vi "Recipe.vi"() -> ()   [LabVIEW 2015]
panel:
  in  "Timer":bool
  in  "Offset":bool
  in  "Speed":bool
  in  "檔案":bool
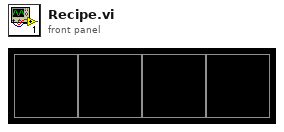
[diagram p1: front panel]
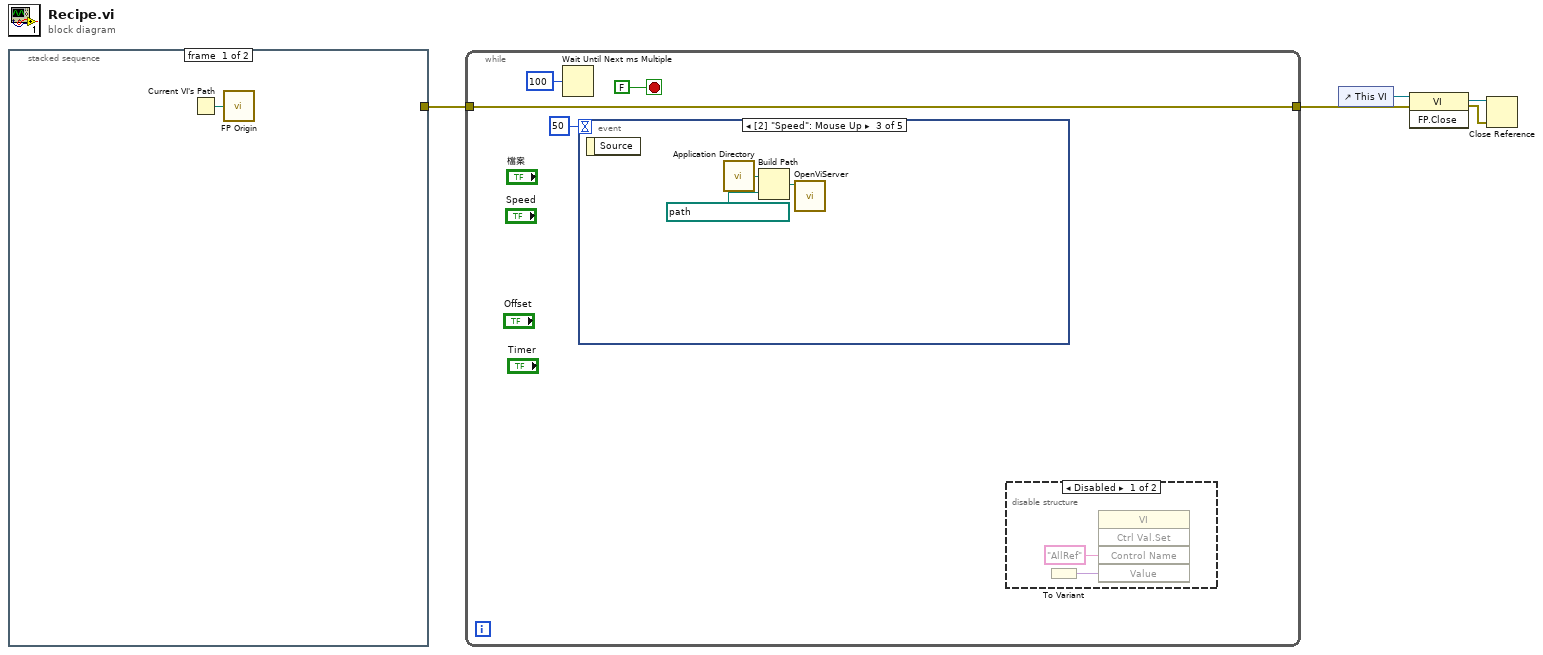
[diagram p0: block diagram]
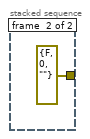
[diagram p2: hidden frame]
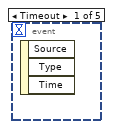
[diagram p4: hidden frame]
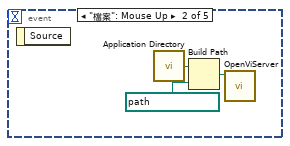
[diagram p5: hidden frame]
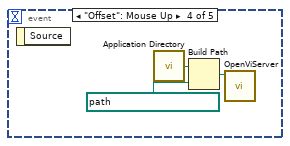
[diagram p6: hidden frame]
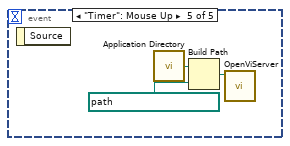
[diagram p7: hidden frame]
diagram:
  n1 = stacked-sequence {
    tunnel: [_ errorcluster {"status"=FALSE, "code"=0, "source"=""} ("error out")] -> w1
    frame #0 {
      n2 = Current VI's Path() -> (path=w6:path)
      n3 = call "FP Origin.vi"("vi path"=w6) -> ()  [unwired: 1 out]
    }
    frame #1 {
    }
  }
  n4 = while {
    tunnel: w1 -> [w9]
    tunnel: [w9] -> w5
    stop <- FALSE stop-if-true
    n5 = Wait Until Next ms Multiple(millisecond multiple=u32 100) -> ()  [unwired: 1 out]
    n6 = event shown="[2] \"Speed\": Mouse Up" {
      selector: _ -> [_ _ _ _ _]
      dyn-events: _ -> [_ _ _ _ _]
      timeout: 50 -> [_ _ _ _ _]
      event Timeout {
        n7 = event-data() -> ()  [unwired: 1 in, 3 out]
      }
      event "檔案": Mouse Up {
        n8 = event-data() -> ()  [unwired: 1 in, 1 out]
        n9 = call <vilib>:"Application Directory.vi"() -> ("Application Directory"=w15:path)
        n10 = Build Path(base path=w15, name or relative path=path "0.Main/檔案.vi" ("vi path")) -> (appended path=w17:path)
        n11 = call "OpenViServer.vi"("vi path"=w17) -> ()  [unwired: 9 in, 2 out]
      }
      event "Speed": Mouse Up {
        n12 = event-data() -> ()  [unwired: 1 in, 1 out]
        n13 = call <vilib>:"Application Directory.vi"() -> ("Application Directory"=w18:path)
        n14 = Build Path(base path=w18, name or relative path=path "0.Main/檔案_速度.vi" ("vi path")) -> (appended path=w20:path)
        n15 = call "OpenViServer.vi"("vi path"=w20) -> ()  [unwired: 9 in, 2 out]
      }
      event "Offset": Mouse Up {
        n16 = event-data() -> ()  [unwired: 1 in, 1 out]
        n17 = call <vilib>:"Application Directory.vi"() -> ("Application Directory"=w21:path)
        n18 = Build Path(base path=w21, name or relative path=path "0.Main/檔案_Offset.vi" ("vi path")) -> (appended path=w23:path)
        n19 = call "OpenViServer.vi"("vi path"=w23) -> ()  [unwired: 9 in, 2 out]
      }
      event "Timer": Mouse Up {
        n20 = event-data() -> ()  [unwired: 1 in, 1 out]
        n21 = call <vilib>:"Application Directory.vi"() -> ("Application Directory"=w24:path)
        n22 = Build Path(base path=w24, name or relative path=path "0.Main/檔案_Timer.vi" ("vi path")) -> (appended path=w26:path)
        n23 = call "OpenViServer.vi"("vi path"=w26) -> ()  [unwired: 9 in, 2 out]
      }
    }
    n24 = disable-structure shown="Disabled" {
      frame Disabled {
        n25 = To Variant() -> (Variant=w13:variant)  [unwired: 1 in]
        n26 = invoke class="VI" method="Ctrl Val.Set"("Control Name"="AllRef", "Value"=w13) -> (error in=w12:errorcluster)  [unwired: 2 in, 5 out]
      }
      frame Enabled {
      }
    }
  }
  n27 = control-ref of="This VI"() -> (w4:refnum<vi>)
  n28 = invoke class="VI" method="FP.Close"(reference=w4, error in=w5) -> (reference out=w3:refnum<vi>, error out=w2:errorcluster)  [unwired: 1 in, 1 out]
  n29 = Close Reference(reference=w3, error in (no error)=w2) -> ()  [unwired: 1 out]
